vi "Unload bitfile.vi"(11 "Session":u32) -> ()   [LabVIEW 2013, in "J1939 Addon Engine.lvlib"]
uses:
  J1939 Addon Engine.lvlib
  NiFpga.dll
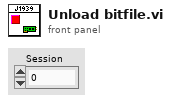
[diagram p1: front panel]
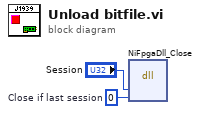
[diagram p0: block diagram]
diagram:
  w2 = u32 0  # Close if last session
  n1 = dll-call lib="NiFpga.dll" fn="NiFpgaDll_Close"("Session"="Session", "Attribute"=w2) -> ()  [unwired: 6 in, 2 out]
